vi "MakeGlobalInvokeRegisterStruct.vi"() -> (3 "Event Registration Refnum out":refnum<event-registration>)   [LabVIEW 2017]
uses:
  Globals/globals.vi
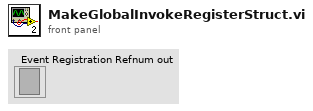
[diagram p1: front panel]
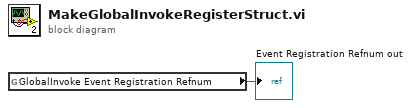
[diagram p0: block diagram]
diagram:
  n1 = global read "globals.vi" "GlobalInvoke Event Registration Refnum"() -> (→"Event Registration Refnum out":refnum<event-registration>)
